vi "Find Fiducial.vi"(4 "Field of View":cluster{"fieldOfViewX":sgl, "fieldOfViewY":sgl}, 5 "Shrink Factor":i32=1, 6 "debug":bool, 8 "error in":errorcluster, 9 "Method Parameters":variant, 10 "Method Name":string, 11 "Image":T2) -> (0 "error out":errorcluster, 1 "log out":string, 2 "Fiducials":T1(array[cluster]))   [LabVIEW 2022 SP3, in "Vision.lvlib"]
uses:
  Vision.lvlib
  find_circles parameters.ctl
  find_patches parameters.ctl
  find_rects_parameters.ctl
  find_template parameters.ctl
  <vilib>/vision/Image Controls.llb/IMAQ Image.ctl
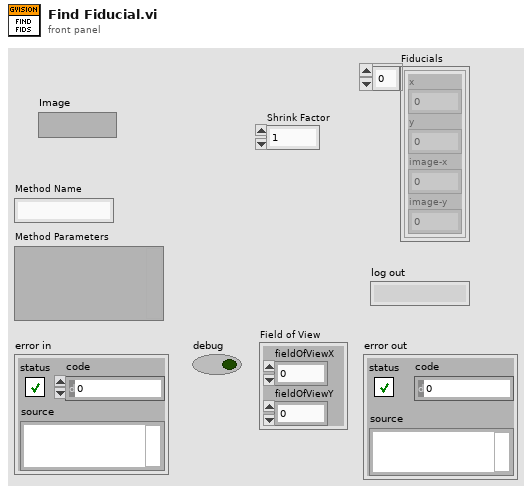
[diagram p1: front panel]
types:
  T1 = cluster{"x":dbl, "y":dbl, "image-x":dbl, "image-y":dbl}[]
  T2 = typedef "IMAQ Image.ctl" = refnum<image>
  T3 = typedef "Vision.lvlib/find_circles parameters.ctl" = cluster{"minRadius":sgl, "maxRadius":sgl, "houghGradientParam1":i32, "houghGradientParam2":i32}
  T4 = cluster{"x":dbl, "y":dbl, "image-x":dbl, "image-y":dbl}
  T5 = typedef "Vision.lvlib/find_patches parameters.ctl" = cluster{"dilateSize":i32, "sizeMin":sgl, "sizeMax":sgl, "aspectRatioMin":sgl, "aspectRatioMax":sgl, "colorGroups":i32}
  T6 = typedef "Vision.lvlib/find_rects_parameters.ctl" = cluster{"nominalWidth":sgl, "nominalHeight":sgl, "tolerance":sgl, "pointSelect":sgl, "allowRotation":bool}
  T7 = typedef "Vision.lvlib/find_template parameters.ctl" = cluster{"templateBlurFactor":i32, "minConcurrence":sgl, "templatePath":string}
  T8 = cluster{"x":dbl, "y":dbl, "radius":dbl, "image-x":dbl, "image-y":dbl}[]
  T9 = cluster{"x":dbl, "y":dbl, "aspect ratio":dbl, "size":dbl, "image-x":dbl, "image-y":dbl}[]
  T10 = cluster{"x":dbl, "y":dbl, "width":dbl, "height":dbl, "angle":dbl, "image-x":dbl, "image-y":dbl}[]
  T11 = cluster{"x":dbl, "y":dbl, "image-x":dbl, "image-y":dbl, "Concurrence":dbl}[]
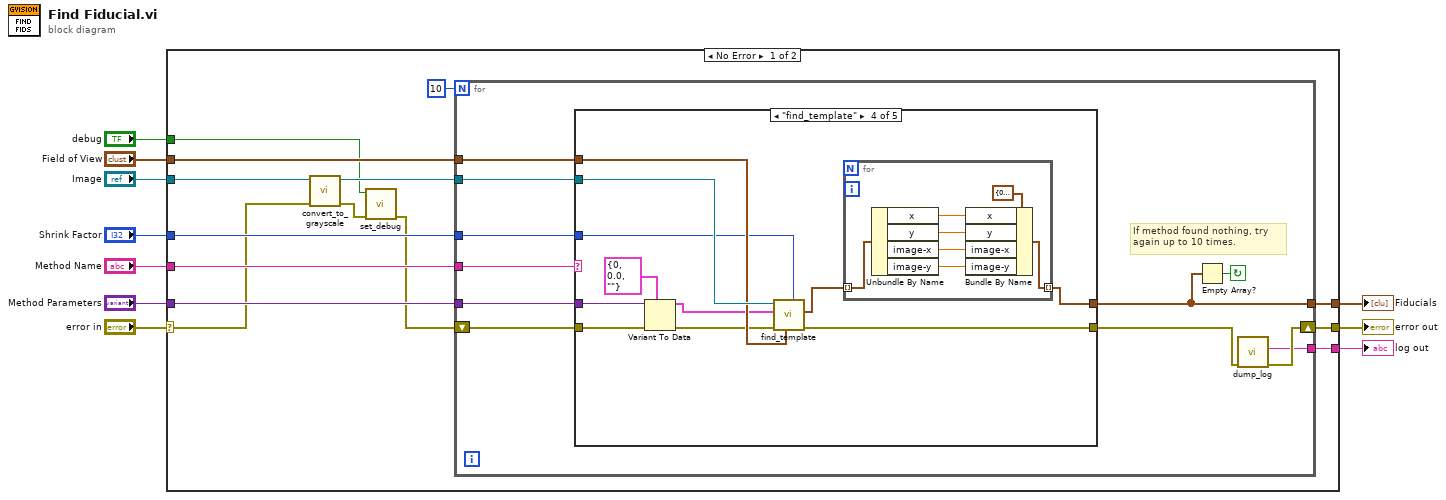
[diagram p0: block diagram]
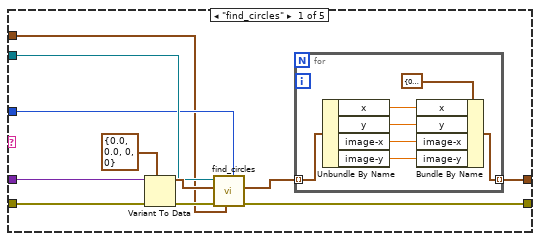
[diagram p2: hidden frame]
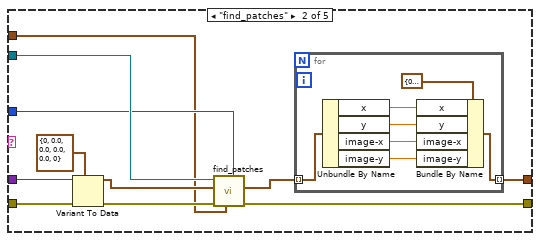
[diagram p3: hidden frame]
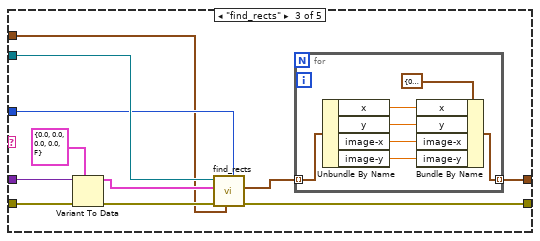
[diagram p4: hidden frame]
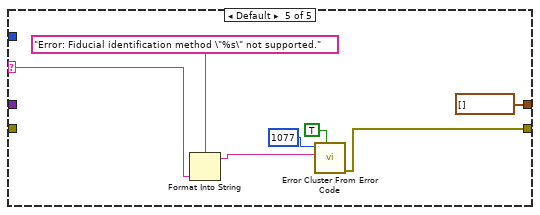
[diagram p5: hidden frame]
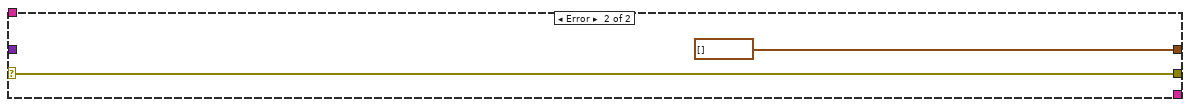
[diagram p6: hidden frame]
diagram:
  n1 = case shown="No Error" "error in" {
    selector: "error in" -> [w15 w116]
    tunnel: [w19 w116] -> w9
    tunnel: "Method Name" -> [w24 _]
    tunnel: "Method Parameters" -> [w23 _]
    tunnel: "Image" -> [w17 _]
    tunnel: "Shrink Factor" -> [w22 _]
    tunnel: "Field of View" -> [w21 _]
    tunnel: "debug" -> [w12 _]
    tunnel: [w20 T1 []] -> w2
    tunnel: [w11 _] -> w1
    frame No Error {
      n2 = call "convert_to_grayscale.vi"("error in (no error)"=w15, "Image in"=w17) -> ("error out"=w14:errorcluster, "Image out"=w16:T2)  [unwired: 8 in]
      n3 = call "set_debug.vi"("error in (no error)"=w14, "debug"=w12) -> ("error out"=w13:errorcluster)  [unwired: 9 in]
      n4 = for {
        N: 10 -> [_]
        tunnel: w24 -> [w35]
        tunnel: w23 -> [w34]
        tunnel: w16 -> [w32]
        tunnel: w22 -> [w31]
        tunnel: w21 -> [w30]
        tunnel: [w29] -> w20
        shift-right: [w26] -> w19
        shift-left: w13 -> [w33]
        tunnel: [w25] -> w11
        stop <- w28 continue-if-true
        # "If method found nothing, try\nagain up to 10 times."
        n5 = case shown="\"find_template\"" w35 {
          selector: w35 -> [_ _ _ _ w112]
          tunnel: w34 -> [w46 w64 w82 w91 _]
          tunnel: w33 -> [w36 w62 w80 w98 _]
          tunnel: w32 -> [w42 w60 w78 w100 _]
          tunnel: w31 -> [w41 w59 w77 w95 _]
          tunnel: w30 -> [w40 w58 w76 w99 _]
          tunnel: [w38 w56 w74 w92 T1 []] -> w29
          tunnel: [w37 w54 w73 w94 w108] -> w27
          frame "find_circles" {
            n6 = Variant To Data(error in=w36, type=T3 {"minRadius"=0.0, "maxRadius"=0.0, "houghGradientParam1"=0, "houghGradientParam2"=0} ("find_circles parameters"), Variant=w46) -> (data=w44:T3, error out=w43:errorcluster)
            n7 = call "find_circles.vi"("shrinkFactor"=w41, "Field of View"=w40, "error in"=w43, "find_circles parameters"=w44, "Image"=w42) -> ("error out"=w37:errorcluster, "Circles"=w39:T8)  [unwired: 5 in]
            n8 = for {
              tunnel: w39 -> [w53] mode=indexing
              tunnel: [w47] -> w38 mode=indexing
              n9 = Unbundle By Name(w53) -> ("x"=w51:dbl, "y"=w50:dbl, "image-x"=w49:dbl, "image-y"=w48:dbl)
              n10 = Bundle By Name(cluster=T4 {"x"=0.0, "y"=0.0, "image-x"=0.0, "image-y"=0.0}, "x"=w51, "y"=w50, "image-x"=w49, "image-y"=w48) -> (w47:T4)
            }
          }
          frame "find_patches" {
            n11 = Variant To Data(error in=w62, type=T5 {"dilateSize"=0, "sizeMin"=0.0, "sizeMax"=0.0, "aspectRatioMin"=0.0, "aspectRatioMax"=0.0, "colorGroups"=0} ("find_patches parameters"), Variant=w64) -> (data=w63:T5, error out=w61:errorcluster)
            n12 = call "find_patches.vi"("Shrink Factor"=w59, "Field of View"=w58, "error in"=w61, "find_patches parameters"=w63, "Image"=w60) -> ("error out"=w54:errorcluster, "Patches"=w57:T9)  [unwired: 5 in]
            n13 = for {
              tunnel: w57 -> [w71] mode=indexing
              tunnel: [w65] -> w56 mode=indexing
              n14 = Unbundle By Name(w71) -> ("x"=w69:dbl, "y"=w68:dbl, "image-x"=w67:dbl, "image-y"=w66:dbl)
              n15 = Bundle By Name(cluster=T4 {"x"=0.0, "y"=0.0, "image-x"=0.0, "image-y"=0.0}, "x"=w69, "y"=w68, "image-x"=w67, "image-y"=w66) -> (w65:T4)
            }
          }
          frame "find_rects" {
            n16 = Variant To Data(error in=w80, type=T6 {"nominalWidth"=0.0, "nominalHeight"=0.0, "tolerance"=0.0, "pointSelect"=0.0, "allowRotation"=FALSE} ("find_patches parameters"), Variant=w82) -> (data=w81:T6, error out=w79:errorcluster)
            n17 = call "find_rects.vi"("shrinkFactor"=w77, "Field of View"=w76, "error in"=w79, "find_patches parameters"=w81, "Image"=w78) -> ("error out"=w73:errorcluster, "rects"=w75:T10)  [unwired: 5 in]
            n18 = for {
              tunnel: w75 -> [w89] mode=indexing
              tunnel: [w83] -> w74 mode=indexing
              n19 = Unbundle By Name(w89) -> ("x"=w87:dbl, "y"=w86:dbl, "image-x"=w85:dbl, "image-y"=w84:dbl)
              n20 = Bundle By Name(cluster=T4 {"x"=0.0, "y"=0.0, "image-x"=0.0, "image-y"=0.0}, "x"=w87, "y"=w86, "image-x"=w85, "image-y"=w84) -> (w83:T4)
            }
          }
          frame "find_template" {
            n21 = Variant To Data(error in=w98, type=T7 {"templateBlurFactor"=0, "minConcurrence"=0.0, "templatePath"=""} ("find_patches parameters"), Variant=w91) -> (data=w90:T7, error out=w97:errorcluster)
            n22 = call "find_template.vi"("Shrink Factor"=w95, "Field of View"=w99, "error in"=w97, "find_template parameters"=w90, "Image"=w100) -> ("error out"=w94:errorcluster, "Matches"=w93:T11)  [unwired: 5 in]
            n23 = for {
              tunnel: w93 -> [w107] mode=indexing
              tunnel: [w101] -> w92 mode=indexing
              n24 = Unbundle By Name(w107) -> ("x"=w105:dbl, "y"=w104:dbl, "image-x"=w103:dbl, "image-y"=w102:dbl)
              n25 = Bundle By Name(cluster=T4 {"x"=0.0, "y"=0.0, "image-x"=0.0, "image-y"=0.0}, "x"=w105, "y"=w104, "image-x"=w103, "image-y"=w102) -> (w101:T4)
            }
          }
          frame Default {
            n26 = Format Into String(format string="Error: Fiducial identification method \"%s\" not supported.", w112) -> (resulting string=w111:string)  [unwired: 2 in, 1 out]
            n27 = call <vilib>:"Error Cluster From Error Code.vi"("show call chain? (False)"=TRUE, "error message (\"\")"=w111, "error code (0)"=1077) -> ("error out"=w108:errorcluster)  [unwired: 6 in]
          }
        }
        n28 = Empty Array?(array=w29) -> (empty?=w28:bool)
        n29 = call "dump_log.vi"("error in (no error)"=w27) -> ("error out"=w26:errorcluster, "log out"=w25:string)  [unwired: 9 in]
      }
    }
    frame Error {
    }
  }
  "error out" <- w9
  "Fiducials" <- w2
  "log out" <- w1
